vi "Extract Data.vi"(8 "error in (no error)":errorcluster caption="entrée d'erreur (pas d'erreur)", 11 "Parsing Data RADIO_ERP1 en entrée":refnum<class "Parsing Data RADIO_ERP1_A5.lvclass">) -> (0 "error out":errorcluster caption="sortie d'erreur", 3 "Parsing Data RADIO_ERP1 en sortie":refnum<class "Parsing Data RADIO_ERP1_A5.lvclass">)   [LabVIEW 2020, in "Library Instrument & Equipement.lvlib" / "Library UART.lvlib" / "Parsing Data RADIO_ERP1_A5.lvclass"]
uses:
  Parsing Data RADIO_ERP1_A5.lvclass
  C:/Users/ngarcin/OneDrive - Altyor/Standard TB/Class/UART/UART Enocean/Parsing Data Enocean (Default)/Parsing Data Enocean (Default).lvclass
  Parsing Data RADIO_ERP1_A5.lvclass/Parsing Data RADIO_ERP1_A5.ctl
  Commun VI/Library Commun.lvlib
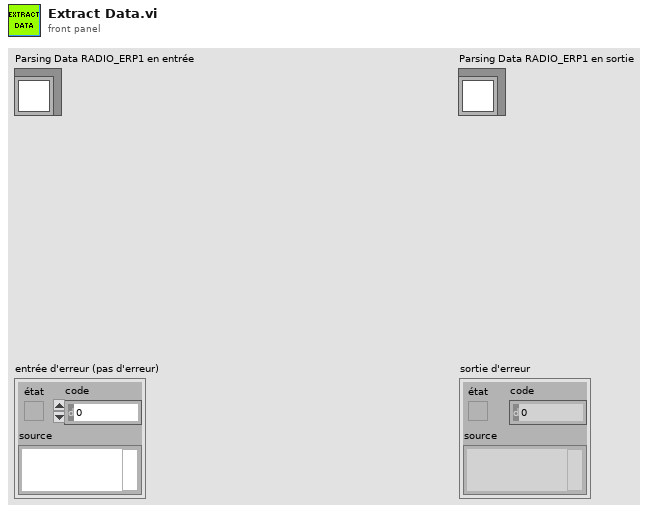
[diagram p1: front panel]
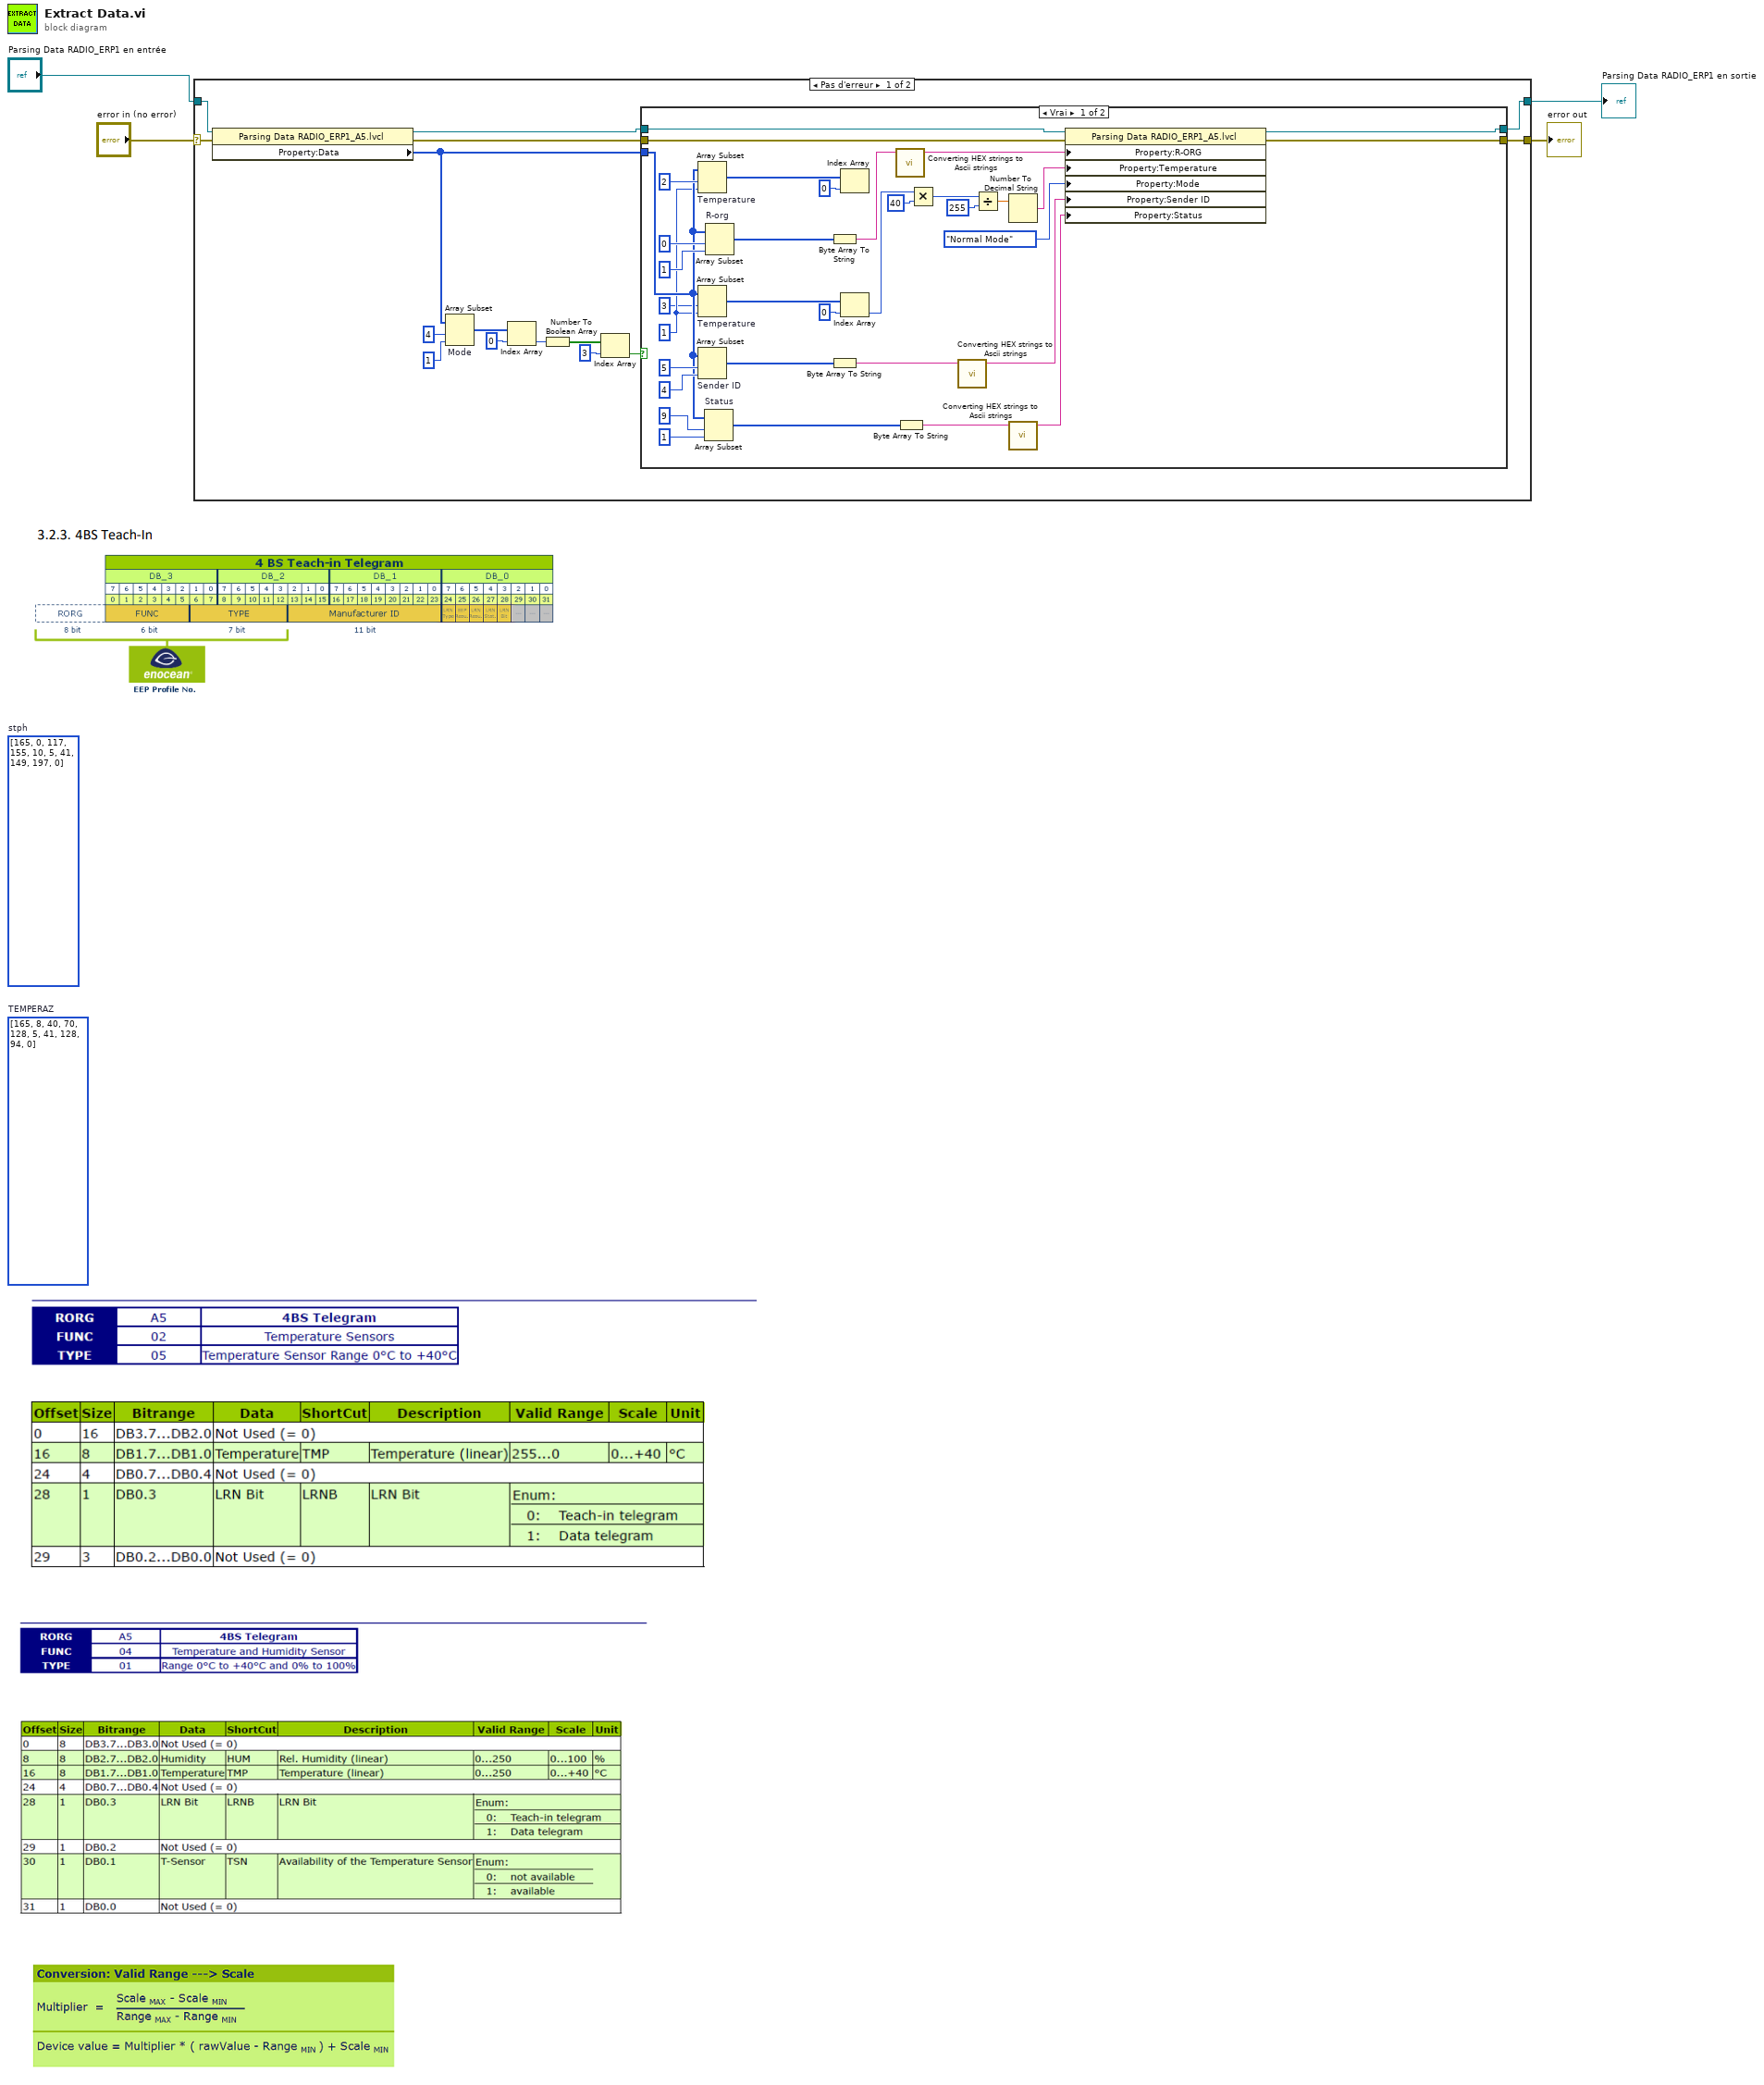
[diagram p0: block diagram]
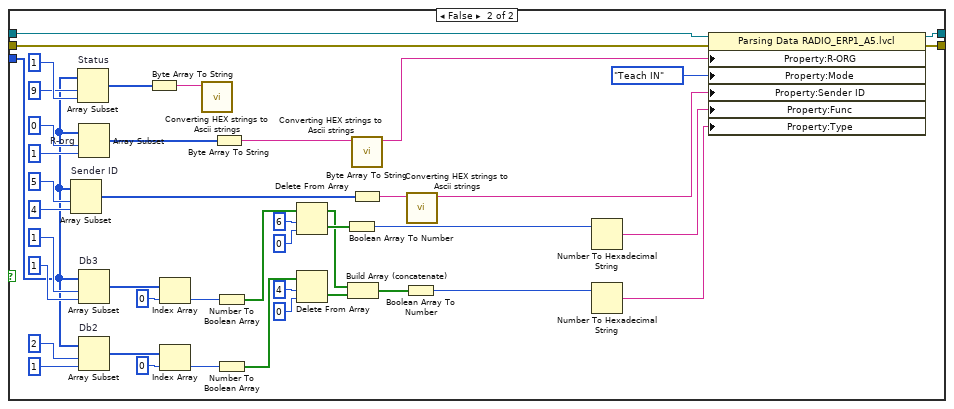
[diagram p2: hidden frame]
diagram:
  (unwired) u8[] [165, 0, 117, 155, 10, 5, 41, 149, 197, 0]  # stph
  (unwired) u8[] [165, 8, 40, 70, 128, 5, 41, 128, 94, 0]  # TEMPERAZ
  n1 = case shown="Pas d'erreur" "error in (no error)" {
    selector: "error in (no error)" -> [w15 w99]
    tunnel: [w14 w99] -> w3
    tunnel: [w16 w98] -> w1
    tunnel: "Parsing Data RADIO_ERP1 en entrée" -> [w17 w98]
    frame No Error {
      n2 = property class="Parsing Data RADIO_ERP1_A5.lvcl"(reference=w17, error in=w15) -> (reference out=w19:refnum<class "Parsing Data RADIO_ERP1_A5.lvclass">, error out=w18:errorcluster, "Property:Data"=w6:u8[])
      n3 = Array Subset "Mode"(array=w6, index=4 ("indice"), length=1 ("longueur")) -> (w11:u8[])
      n4 = Index Array(array=w11, index=0 ("indice")) -> (element=w7:u8)
      n5 = Number To Boolean Array(number=w7) -> (Boolean array=w9:bool[])
      n6 = Index Array(array=w9, index=3 ("indice")) -> (element=w5:bool)
      n7 = case shown="Vrai" w5 {
        tunnel: w19 -> [w53 w97]
        tunnel: w18 -> [w42 w87]
        tunnel: [w41 w86] -> w16
        tunnel: [w40 w85] -> w14
        tunnel: w6 -> [w28 w65]
        frame True {
          w27 = 1 ("longueur")
          n8 = Array Subset "Temperature"(array=w28, index=2 ("indice"), length=w27) -> (w33:u8[])
          n9 = Array Subset "Temperature"(array=w28, index=3 ("indice"), length=w27) -> (w24:u8[])
          n10 = Array Subset "Sender ID"(array=w28, index=5 ("indice"), length=4 ("longueur")) -> (w48:u8[])
          n11 = Array Subset "Status"(array=w28, index=9 ("indice"), length=1 ("indice")) -> (w43:u8[])
          n12 = Array Subset "R-org"(array=w28, index=0 ("indice"), length=1 ("longueur")) -> (w51:u8[])
          n13 = Byte Array To String(unsigned byte array=w51) -> (string=w50:string)
          n14 = Byte Array To String(unsigned byte array=w48) -> (string=w47:string)
          n15 = Index Array(array=w33, index=0 ("indice")) -> ()  [unwired: 1 out]
          n16 = Index Array(array=w24, index=0 ("indice")) -> (element=w23:u8)
          n17 = call "Converting HEX strings to Ascii strings.vi"("chaîne IN"=w50) -> ("Chaîne OUT"=w49:string)  [unwired: 9 in, 1 out]
          n18 = Byte Array To String(unsigned byte array=w43) -> (string=w45:string)
          n19 = Multiply(x=w23, y=u16 40 ("x")) -> (x*y=w21:u16)
          n20 = call "Converting HEX strings to Ascii strings.vi"("chaîne IN"=w47) -> ("Chaîne OUT"=w46:string)  [unwired: 9 in, 1 out]
          n21 = Divide(x=w21, y=u16 255) -> (x/y=w20:dbl)
          n22 = Number To Decimal String(number=w20) -> (decimal integer string=w32:string)  [unwired: 1 in]
          n23 = call "Converting HEX strings to Ascii strings.vi"("chaîne IN"=w45) -> ("Chaîne OUT"=w44:string)  [unwired: 9 in, 1 out]
          n24 = property class="Parsing Data RADIO_ERP1_A5.lvcl"(reference=w53, error in=w42, "Property:R-ORG"=w49, "Property:Temperature"=w32, "Property:Mode"=enum16{"Teach IN", "Normal Mode"}."Normal Mode" ("Mode"), "Property:Sender ID"=w46, "Property:Status"=w44) -> (reference out=w41:refnum<class "Parsing Data RADIO_ERP1_A5.lvclass">, error out=w40:errorcluster)
        }
        frame False {
          n25 = Array Subset "Sender ID"(array=w65, index=5 ("indice"), length=4 ("longueur")) -> (w92:u8[])
          n26 = Array Subset "Status"(array=w65, index=9 ("indice"), length=1 ("indice")) -> (w88:u8[])
          n27 = Array Subset "R-org"(array=w65, index=0 ("indice"), length=1 ("longueur")) -> (w95:u8[])
          n28 = Array Subset "Db3"(array=w65, index=1 ("indice"), length=1 ("longueur")) -> (w76:u8[])
          n29 = Array Subset "Db2"(array=w65, index=2 ("indice"), length=1 ("longueur")) -> (w64:u8[])
          n30 = Byte Array To String(unsigned byte array=w88) -> (string=w89:string)
          n31 = Index Array(array=w76, index=0 ("indice")) -> (element=w74:u8)
          n32 = Index Array(array=w64, index=0 ("indice")) -> (element=w63:u8)
          n33 = call "Converting HEX strings to Ascii strings.vi"("chaîne IN"=w89) -> ()  [unwired: 9 in, 2 out]
          n34 = Byte Array To String(unsigned byte array=w95) -> (string=w94:string)
          n35 = Number To Boolean Array(number=w74) -> (Boolean array=w73:bool[])
          n36 = Number To Boolean Array(number=w63) -> (Boolean array=w62:bool[])
          n37 = Delete From Array(array=w73, length=6 ("longueur"), index=0 ("indice")) -> (deleted portion=w71:bool[], array with subset deleted=w60:bool[])
          n38 = Delete From Array(array=w62, length=4 ("longueur"), index=0 ("indice")) -> (deleted portion=w59:bool[])  [unwired: 1 out]
          n39 = Boolean Array To Number(Boolean array=w71) -> (number=w70:u32)
          n40 = Build Array (concatenate)(w60, w59) -> (w57:bool[])
          n41 = call "Converting HEX strings to Ascii strings.vi"("chaîne IN"=w94) -> ("Chaîne OUT"=w93:string)  [unwired: 9 in, 1 out]
          n42 = Byte Array To String(unsigned byte array=w92) -> (string=w91:string)
          n43 = Boolean Array To Number(Boolean array=w57) -> (number=w58:u32)
          n44 = call "Converting HEX strings to Ascii strings.vi"("chaîne IN"=w91) -> ("Chaîne OUT"=w90:string)  [unwired: 9 in, 1 out]
          n45 = Number To Hexadecimal String(2:w70) -> (0:w69:string)  [unwired: 1 in]
          n46 = Number To Hexadecimal String(2:w58) -> (0:w56:string)  [unwired: 1 in]
          n47 = property class="Parsing Data RADIO_ERP1_A5.lvcl"(reference=w97, error in=w87, "Property:R-ORG"=w93, "Property:Mode"=enum16{"Teach IN", "Normal Mode"}."Teach IN" ("Mode"), "Property:Sender ID"=w90, "Property:Func"=w69, "Property:Type"=w56) -> (reference out=w86:refnum<class "Parsing Data RADIO_ERP1_A5.lvclass">, error out=w85:errorcluster)
        }
      }
    }
    frame Error {
    }
  }
  "error out" <- w3
  "Parsing Data RADIO_ERP1 en sortie" <- w1
